vi "Read Key (Boolean).vi"(7 "section":string caption="Abschnitt", 8 "error in (no error)":errorcluster caption="Fehler (Eingang, kein Fehler)", 9 "default value":bool caption="Standardwert", 10 "key":string caption="Schlüssel", 11 "refnum":T1 caption="RefNum") -> (0 "error out":errorcluster caption="Fehler (Ausgang)", 1 "value":bool caption="Wert", 2 "found?":bool caption="Gefunden?", 3 "refnum out":T1 caption="RefNum (Ausgang)")   [LabVIEW 2009]
doc: "Liest einen Wert, der einem Schlüssel in einem angegebenen Abschnitt in der durch <B>Refnum</B> angegebenen Konfigurationsdatei zugeordnet ist. Wenn der Schlüssel nicht existiert, wird vom VI der Standardwert ausgegeben. Mit diesem polymorphen VI können folgende Wertetypen aus einem Schlüssel ausgelesen werden: boolesche Werte, numerische Werte mit doppelter Genauigkeit, vorzeichenbehaftete Integer-Werte, Pfade, Strings und vorzeichenlose Integer-Werte. Durch den Datentyp, der am Eingang <B>Index</B> anliegt, wird die zu verwendende Instanz des polymorphen VIs festgelegt."
uses:
  <vilib>/Utility/config.llb/Config Data RefNum.ctl
  <vilib>/Utility/config.llb/NI_LVConfig.lvlib
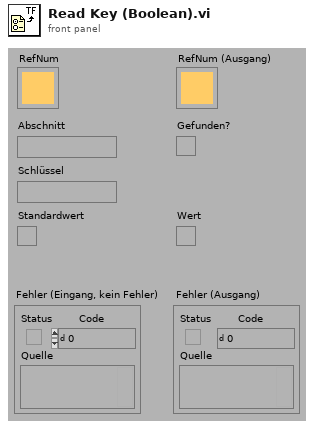
[diagram p1: front panel]
types:
  T1 = typedef "NI_LVConfig.lvlib/Config Data RefNum.ctl" = refnum<k1>
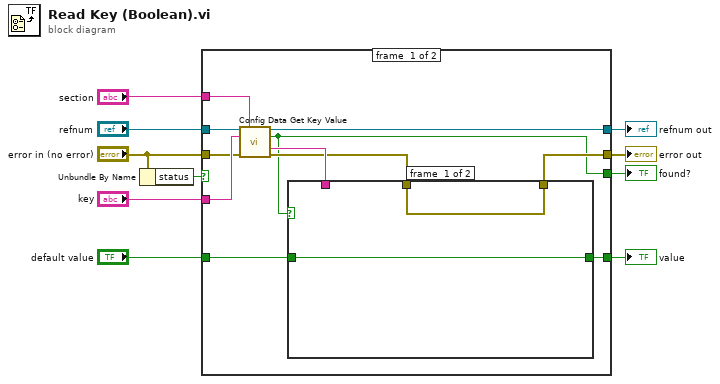
[diagram p0: block diagram]
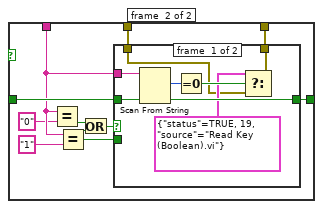
[diagram p2: hidden frame]
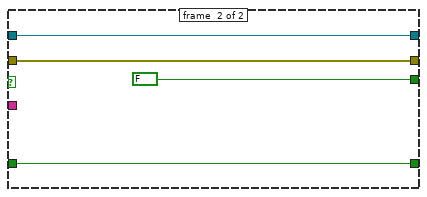
[diagram p4: hidden frame]
diagram:
  n1 = Unbundle By Name("error in (no error)") -> ("status"=w10:bool)
  n2 = case shown="False" w10 {
    tunnel: [w18 w46] -> w4
    tunnel: [w12 w47] -> w1
    tunnel: "refnum" -> [w16 w46]
    tunnel: "error in (no error)" -> [w17 w47]
    tunnel: "section" -> [w21 _]
    tunnel: "key" -> [w20 _]
    tunnel: [w11 FALSE ("section exists?")] -> w3
    tunnel: [w19 w45] -> w2
    tunnel: "default value" -> [w15 w45]
    frame #0 {
      n3 = call "Config Data Get Key Value.vi"("config data"=w16, "section"=w21, "key"=w20, "error in (no error)"=w17) -> ("config data out"=w18:T1, "key exists?"=w11:bool, "key value"=w14:string, "error out"=w13:errorcluster)  [unwired: 6 in, 2 out]
      n4 = case shown="True" w11 {
        tunnel: [w23 w33] -> w19
        tunnel: w15 -> [w23 w32]
        tunnel: w14 -> [_ w31]
        tunnel: w13 -> [w22 w25]
        tunnel: [w22 w24] -> w12
        frame #0 {
        }
        frame #1 {
          n5 = Equal?(x=w31, y="0") -> (x = y?=w27:bool)
          n6 = Equal?(x=w31, y="1") -> (x = y?=w28:bool)
          n7 = Or(x=w27, y=w28) -> (x .or. y?=w26:bool)
          n8 = case shown="False" w26 {
            tunnel: [w41 w43] -> w33
            tunnel: w31 -> [w40 _]
            tunnel: w32 -> [w39 _]
            tunnel: w28 -> [_ w43]
            tunnel: w25 -> [w34 w42]
            tunnel: [w36 w42] -> w24
            frame #0 {
              n9 = Scan From String(input string=w40, default 1=w39) -> (offset past scan=w38:u32, output 1=w41:bool)  [unwired: 3 in, 2 out]
              n10 = Equal To 0?(x=w38) -> (x = 0?=w37:bool)
              n11 = Select(t=cluster{"status":bool, u16, "source":string} {"status"=TRUE, 19, "source"="Read Key (Boolean).vi"} ("f"), s=w37, f=w34) -> (s? t:f=w36:errorcluster)
            }
            frame #1 {
            }
          }
        }
      }
    }
    frame #1 {
    }
  }
  "error out" <- w1
  "refnum out" <- w4
  "value" <- w2
  "found?" <- w3
